vi "Read Msg Output.vi"(11 "TEMPLATE Msg Output in":refnum<class "TEMPLATE Msg Output.lvclass">) -> ()   [LabVIEW 2025, in "_Template.lvlib" / "Templates.lvlib" / "TEMPLATE Msg.lvlib" / "TEMPLATE Msg Output.lvlib" / "TEMPLATE Msg Output.lvclass"]
uses:
  TEMPLATE Msg Output.lvclass
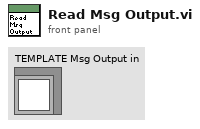
[diagram p1: front panel]
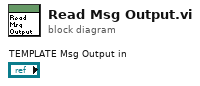
[diagram p0: block diagram]
diagram:
